vi "PH_Sequencer_Watch.PC _PPMeasVolt.vi"(0 "i ref in":refnum<vi>, 2 "Tagname":string, 3 "Tagvalue":dbl, 4 "no link":bool, 5 "error in (no error)":errorcluster) -> (14 "i ref out":refnum<vi>, 19 "error out":errorcluster)   [LabVIEW 2014, in "PH_Sequencer_Watch.lvlib"]
doc: "This VI writes the incoming information for measured voltage to the related GUI element and to own attributes."
uses:
  PH_Sequencer_Watch.lvlib
  PH_Beckhoff_PP_PU/PH_Beckhoff_PP_PU.HV Meas Tags.ctl
  PH_Beckhoff_PP_PU/PH_Beckhoff_PP_PU.lvlib
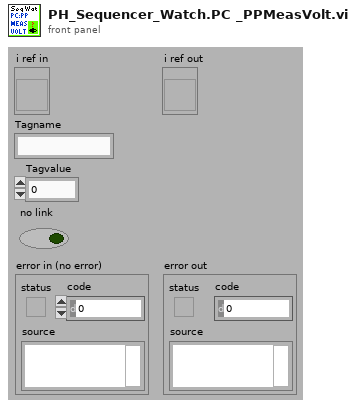
[diagram p1: front panel]
types:
  T1 = typedef "PH_Sequencer_Watch.lvlib/PH_Sequencer_Watch.i attribute.ctl" = cluster{"GUI Refs":cluster{"Shot ID":refnum<vi>, "Sequencer SM State":refnum<vi>, "Remaining Time":refnum<vi>, "PHELIX_Timing_T2":refnum<vi>, "T2-Unit-Dummy":refnum<vi>, "fs_Synchrolock_Watch":refnum<vi>, "Experiment_Vacuum_Control_Experiment":refnum<vi>}, "Status Synchrolock":T2, "Exp - Pressure":dbl, "Exp - Limit":dbl, "Heads":T3[], "Refs BooleanState":refnum<vi>[]}
  T2 = typedef "PH_StatusHandler.lvlib/PH_StatusHandler.Status.ctl" = i16
  T3 = typedef "PH_Sequencer_Watch.lvlib/PH_Sequencer_Watch.Head Information.ctl" = cluster{"Ref Volt":refnum<vi>, "PU":T4}
  T4 = typedef "PH_PP_Common.lvlib/PH_PP_Common.PUs.ctl" = enum16{"no Info", "PA-19mm-1", "PA-19mm-2", "PA-45mm-PILC", "PA-45mm-MAIN", "MA-PU-1", "MA-PU-2", "MA-PU-3", "MA-PU-4", "MA-PU-5", "MA-PU-6", "MA-FR", "MA-PILC", "PA-45mm-DP"}
  T5 = typedef "PH_Beckhoff_PP_PU.lvlib/PH_Beckhoff_PP_PU.HV Meas Tags.ctl" = enum16{"voltage-raw", "voltage"}
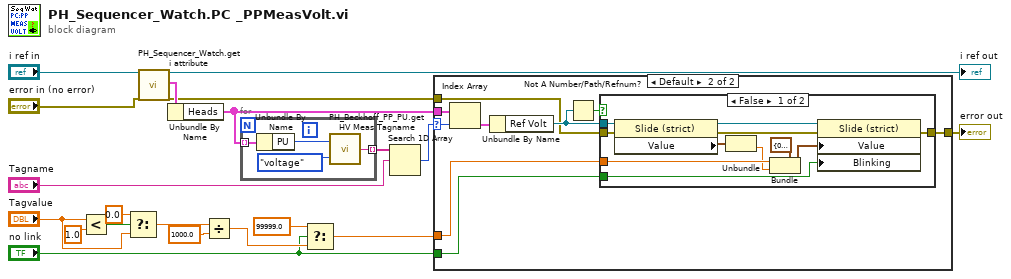
[diagram p0: block diagram]
diagram:
  n1 = Less?(x="Tagvalue", y=1.0) -> (x < y?=w15:bool)
  n2 = Select(t=0.0, s=w15, f="Tagvalue") -> (s? t:f=w8:dbl)
  n3 = call "PH_Sequencer_Watch.get i attribute.vi"("i ref in"="i ref in", "error in (no error)"="error in (no error)") -> ("i ref out"=→"i ref out":refnum<vi>, "i attribute"=w17:T1, "error out"=w5:errorcluster)  [unwired: 15 in]
  n4 = Unbundle By Name(w17) -> ("Heads"=w4:T3[])
  n5 = Divide(x=w8, y=1000.0) -> (x/y=w9:dbl)
  n6 = for {
    tunnel: w4 -> [w24] mode=indexing
    tunnel: [w22] -> w3 mode=indexing
    n7 = Unbundle By Name(w24) -> ("PU"=w23:T4)
    n8 = call "PH_Beckhoff_PP_PU.get HV Meas Tagname.vi"("HV Meas Tag"=PH_Beckhoff_PP_PU.HV_Meas_Tags."voltage", "PU"=w23) -> ("HV Meas Tagname"=w22:string)
  }
  n9 = Select(t=99999.0, s="no link", f=w9) -> (s? t:f=w11:dbl)
  n10 = Search 1D Array(1D array=w3, element="Tagname") -> (index of element=w1:i32)  [unwired: 1 in]
  n11 = case shown="Default" w1 {
    selector: w1 -> [_ w28]
    tunnel: [w25 w34] -> w12
    tunnel: w11 -> [_ w33]
    tunnel: "no link" -> [_ w32]
    tunnel: w5 -> [w25 w27]
    tunnel: w4 -> [_ w31]
    frame -1 {
    }
    frame Default {
      n12 = Index Array(array=w31, index=w28) -> (element=w30:T3)
      n13 = Unbundle By Name(w30) -> ("Ref Volt"=w29:refnum<vi>)
      n14 = Not A Number/Path/Refnum?(number/path/refnum=w29) -> (NaN/Path/Refnum?=w26:bool)
      n15 = case shown="False" w26 {
        tunnel: w29 -> [w39 _]
        tunnel: w27 -> [w44 w46]
        tunnel: [w43 w46] -> w34
        tunnel: w33 -> [w42 _]
        tunnel: w32 -> [w40 _]
        frame False {
          n16 = property class="Slide (strict)"(reference=w39, error in=w44) -> (reference out=w41:refnum<vi>, error out=w45:errorcluster, "Value"=w38:cluster{dbl, dbl})
          n17 = Unbundle(w38) -> (w35:dbl)  [unwired: 1 out]
          n18 = Bundle(cluster=cluster{dbl, dbl} {0.0, 0.0} ("Value"), w42, w35) -> (w37:cluster{dbl, dbl})
          n19 = property class="Slide (strict)"(reference=w41, error in=w45, "Value"=w37, "Blinking"=w40) -> (error out=w43:errorcluster)  [unwired: 1 out]
        }
        frame True {
        }
      }
    }
  }
  "error out" <- w12
